vi "NI VeriStand - Get Item Reference by Path.vi"(8 "error in (no error)":errorcluster, 10 "Root Ref":T1=18446744073709551615 format="%.0x", 11 "Item Path in":string) -> (0 "error out":errorcluster, 2 "Item Ref":T1 format="%.0x", 3 "Item Path out":string, 4 "Found":bool)   [LabVIEW 2020, in "Custom Device API.lvlib"]
doc: "Returns a reference to the custom device item specified by <B>Item Path in</B>."
uses:
  <vilib>/NI VeriStand/Custom Device API/Custom Device API.lvlib
  <vilib>/NI VeriStand/Custom Device API/Custom Device Item Ref.ctl
  07a2599a-e5c4-4b81-bc15-983493d62f68.vi
  <vilib>/NI VeriStand/Custom Device API/Custom Device Offline Path.vi
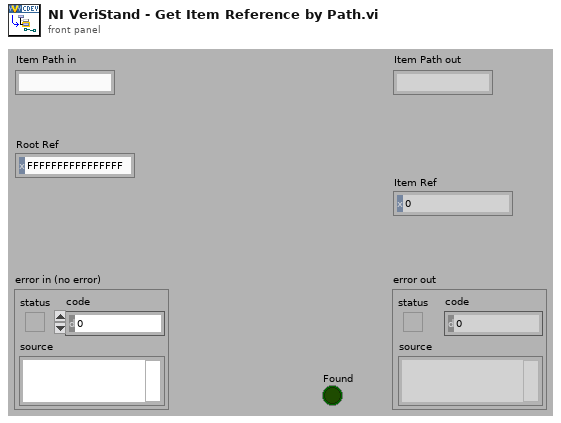
[diagram p1: front panel]
types:
  T1 = typedef "Custom Device API.lvlib/Custom Device Item Ref.ctl" = u64
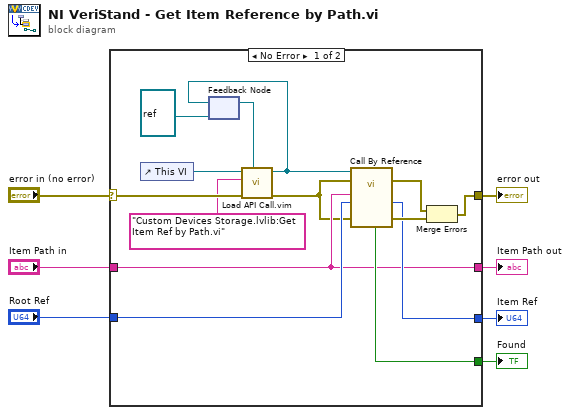
[diagram p0: block diagram]
diagram:
  n1 = case shown="No Error" "error in (no error)" {
    selector: "error in (no error)" -> [w13 w23]
    tunnel: [w20 w23] -> w7
    tunnel: "Item Path in" -> [w16 w22]
    tunnel: [w16 w22] -> w5
    tunnel: [w19 _] -> w4
    tunnel: [w18 _] -> w3
    tunnel: "Root Ref" -> [w17 _]
    frame No Error {
      n2 = control-ref of="This VI"() -> (w14:refnum<vi>)
      n3 = feedback #1(refnum<vi> refnum ("type specifier VI Refnum (for type only)")) -> (w15:refnum<vi>)
      n4 = call "Load API Call.vim"("VI reference in"=w15, "error in (no error)"=w13, "VI qualified name"="Custom Devices Storage.lvlib:Get Item Ref by Path.vi", "Caller VI ref"=w14) -> ("error out"=w12:errorcluster, "VI reference"=w11:refnum<vi>)  [unwired: 6 in]
      n5 = feedback-in #1(w11) -> ()
      n6 = call-by-ref "?"(reference=w11, error in=w12, 8:"error in (no error)"=w12, "Root Ref"=w17, "Item Path in"=w16) -> (error out=w8:errorcluster, 0:"error out"=w21:errorcluster, "Item Ref"=w19:T1, "Found"=w18:bool)  [unwired: 5 in, 2 out]
      n7 = Merge Errors(w8, w21) -> (w20:errorcluster)
    }
    frame Error {
    }
  }
  "error out" <- w7
  "Found" <- w3
  "Item Ref" <- w4
  "Item Path out" <- w5
